vi "FrontPanelToIni.vi"(8 "ErrorArray In":errorcluster[](array[cluster])) -> (0 "ErrorArray Out":errorcluster[](array[cluster]))   [LabVIEW 2014, in "Framework.lvlib"]
uses:
  Framework.lvlib
  <vilib>/Utility/config.llb/Config Data RefNum.ctl
  Config_class/Config.lvclass/Config.ctl
  TypeDefs/clInitParams.ctl
  Config_class/Typedefs/eLogLvl.ctl
  Config_class/Accessors/Read ConfigFilePath.vi
  Config_class/Read Logging.vi
  Config_class/Accessors/Read PARTF Root Directory.vi
  <vilib>/Utility/error.llb/Error Cluster From Error Code.vi
  <vilib>/ErrorRing/Error Ring.xnode
  <userlib>/NIST/NISTErrorLib/NISTErrorLib.lvlib
  <vilib>/Utility/config.llb/NI_LVConfig.lvlib
  Config_class/Config.lvclass
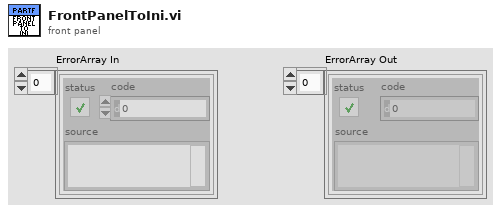
[diagram p1: front panel]
types:
  T1 = typedef "NI_LVConfig.lvlib/Config Data RefNum.ctl" = refnum<k1>
  T2 = typedef "Framework.lvlib/clInitParams.ctl" = cluster{"RowHdrs":string[], "ColHdrs":string[], "DefaultParams":string[][]}
  T3 = typedef "Framework.lvlib/clFrontPanelControlRefs.ctl" = cluster{"TestFilePathRef":refnum<vi>, "BusNumberRef":refnum<vi>, "NumberOfBusesRef":refnum<vi>, "EvtTypeRef":refnum<vi>, "EvtParamsRef":refnum<vi>, "EvtConfigRef":refnum<vi>, "StartTimeRef":refnum<vi>, "EndTimeRef":refnum<vi>, "PmuImpairTypeRef":refnum<vi>, "PmuImpairParamsRef":refnum<vi>, "NetImpairParamsRef":refnum<vi>, "FlagImpairTypeRef":refnum<vi>, "FlagImpairParamsRef":refnum<vi>, "NetImpairTypeRef":refnum<vi>, "OutputFileType":refnum<vi>, "PmuImpairConfigRef":refnum<vi>, "AppTypeRef":refnum<vi>, "ScriptPathRef":refnum<vi>, "ShowPanels?":refnum<vi>}
  T4 = typedef "Framework.lvlib/clEventConfig.ctl" = cluster{"UTC Time 0":timestamp, "Nominal Frequency":u16, "Reporting Rate":u16, "Fsamp":u32, "PosSeq":bool}
  T5 = typedef "PmuImpairPlugins.lvlib/PmuImpairPluginBase.lvclass/clImpairConfig.ctl" = cluster{"FilterType":string, "bPosSeq":bool}
  T6 = typedef "Framework.lvlib/Config.lvclass/eLogLvl.ctl" = enum16{"Normal", "Verbose", "None"}
  T7 = cluster{"pathRootDir":path, "OutDir":string, "ScriptDir":string, "TestDir":string}
  T8 = typedef "Framework.lvlib/Config.lvclass/Logging.ctl" = cluster{"eLogLvl":T6, "Log File Path":path, "btnLogFile":bool}
  T9 = typedef "Framework.lvlib/Config.lvclass/RootDir.ctl" = cluster{"pathRootDir":path, "btnOutPath":bool, "OutDir":string, "btnOpenOutputDir":bool, "ScriptDir":string, "btnOpenScriptDir":bool, "TestDir":string, "btnOpenTestDir":bool}
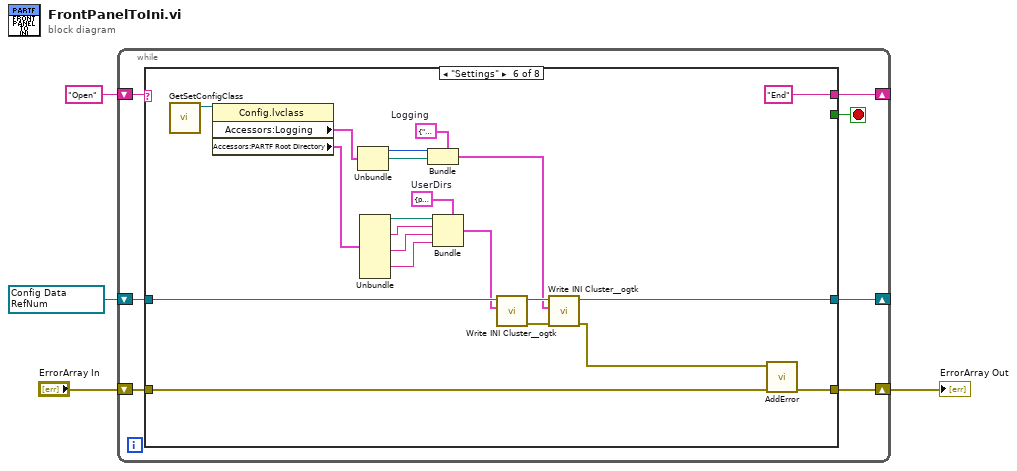
[diagram p0: block diagram]
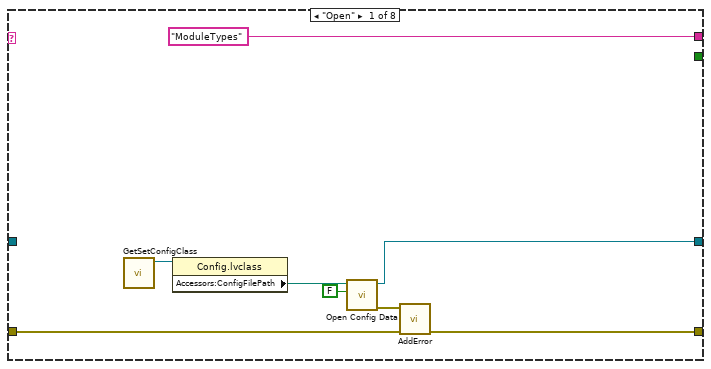
[diagram p2: hidden frame]
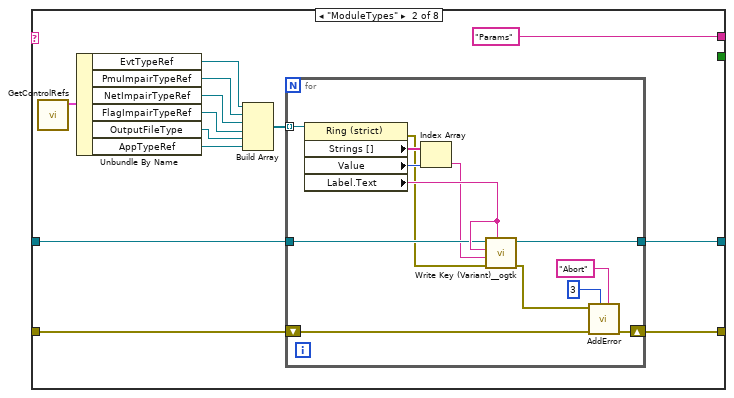
[diagram p3: hidden frame]
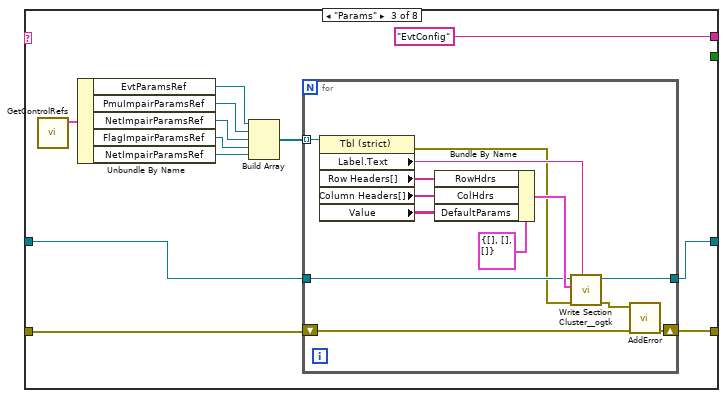
[diagram p4: hidden frame]
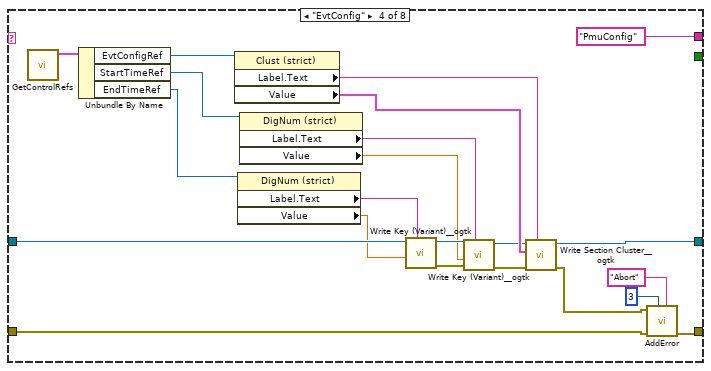
[diagram p5: hidden frame]
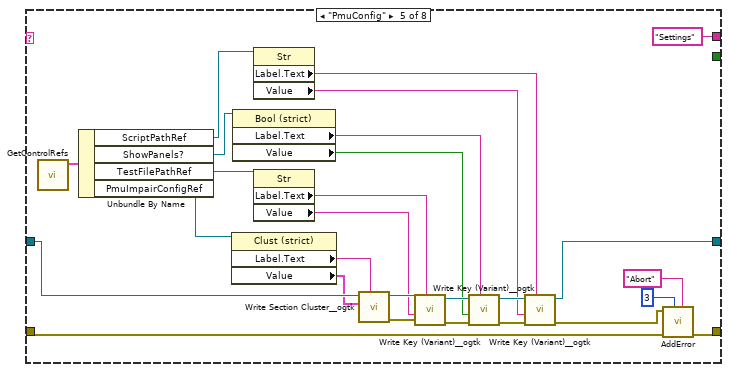
[diagram p6: hidden frame]
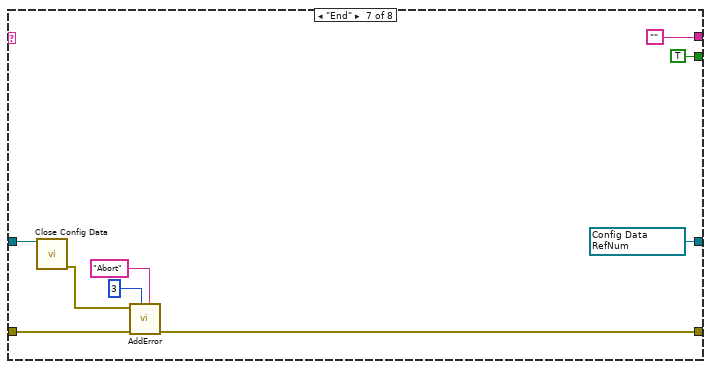
[diagram p7: hidden frame]
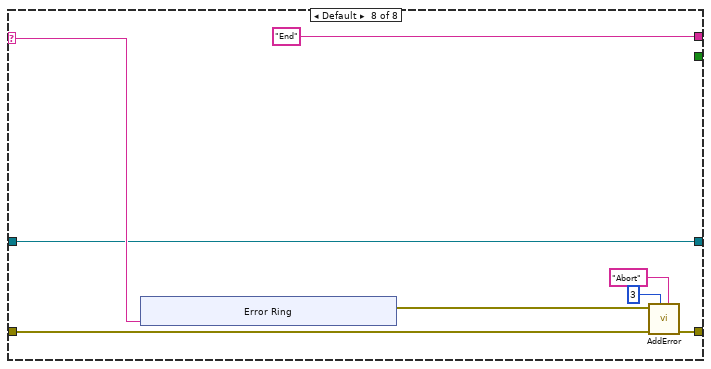
[diagram p8: hidden frame]
diagram:
  w1 = T1 refnum items=["config data"] ("refnum")
  n1 = while {
    shift-right: [w9] -> w2
    shift-left: "ErrorArray In" -> [w10]
    shift-right: [w8] -> _
    shift-left: w1 -> [w6]
    shift-right: [w7] -> _
    shift-left: "Open" -> [w11]
    stop <- w5 stop-if-true
    n2 = case shown="\"Settings\"" w11 {
      selector: w11 -> [_ _ _ _ _ _ _ w157]
      tunnel: w10 -> [w14 w23 w47 w71 w96 w122 w145 w153]
      tunnel: [w13 w22 w48 w75 w98 w123 w144 w152] -> w9
      tunnel: [w16 w21 w49 w76 w93 w124 w141 w150] -> w8
      tunnel: ["ModuleTypes" "Params" "EvtConfig" "PmuConfig" "Settings" "End" "" "End"] -> w7
      tunnel: w6 -> [_ w24 w50 w84 w116 w129 w147 w150]
      tunnel: [_ _ _ _ _ _ TRUE _] -> w5
      frame "Open" {
        n3 = call "GetSetConfigClass.vi"() -> ("Ref out"=w19:refnum<class "Config.lvclass">)  [unwired: 11 in]
        n4 = property class="Config.lvclass"(reference=w19) -> ("Accessors:ConfigFilePath"=w18:path)  [unwired: 1 in, 2 out]
        n5 = call <vilib>:"Open Config Data.vi"("create file if necessary (T)"=FALSE, "configuration file path"=w18) -> ("error out"=w15:errorcluster, "refnum"=w16:T1)  [unwired: 7 in, 1 out]
        n6 = call <userlib>:"AddError.vi"("ErrorArray"=w14, "error in (no error)"=w15) -> ("ErrorArray"=w13:errorcluster[])  [unwired: 8 in, 1 out]
      }
      frame "ModuleTypes" {
        n7 = call "GetControlRefs.vi"() -> ("clControlRefs Out"=w32:T3)  [unwired: 11 in]
        n8 = Unbundle By Name(w32) -> ("EvtTypeRef"=w26:refnum<vi>, "PmuImpairTypeRef"=w27:refnum<vi>, "NetImpairTypeRef"=w28:refnum<vi>, "FlagImpairTypeRef"=w29:refnum<vi>, "OutputFileType"=w30:refnum<vi>, "AppTypeRef"=w31:refnum<vi>)
        n9 = Build Array(w26, w27, w28, w29, w30, w31) -> (w25:refnum<vi>[])
        n10 = for {
          tunnel: w25 -> [w45] mode=indexing
          tunnel: w24 -> [w43]
          shift-right: [w36] -> w22
          shift-left: w23 -> [w37]
          tunnel: [w35] -> w21
          n11 = property class="Ring (strict)"(reference=w45) -> (error out=w33:errorcluster, "Strings []"=w42:string[], "Value"=w41:u16, "Label.Text"=w44:string)  [unwired: 1 in, 1 out]
          n12 = Index Array(array=w42, index=w41) -> (element=w40:string)
          n13 = call <userlib>:"Write Key (Variant)__ogtk.vi"("section"=w44, "error in (no error)"=w33, "key-value"=w40, "key (optional)"=w44, "refnum"=w43) -> ("error out"=w34:errorcluster, "refnum out"=w35:T1)  [unwired: 5 in]
          n14 = call <userlib>:"AddError.vi"("Severity"="Abort", "Priority"=u8 3, "ErrorArray"=w37, "error in (no error)"=w34) -> ("ErrorArray"=w36:errorcluster[])  [unwired: 6 in, 1 out]
        }
      }
      frame "Params" {
        n15 = call "GetControlRefs.vi"() -> ("clControlRefs Out"=w52:T3)  [unwired: 11 in]
        n16 = Unbundle By Name(w52) -> ("EvtParamsRef"=w57:refnum<vi>, "PmuImpairParamsRef"=w56:refnum<vi>, "NetImpairParamsRef"=w55:refnum<vi>, "FlagImpairParamsRef"=w54:refnum<vi>, "NetImpairParamsRef"=w53:refnum<vi>)
        n17 = Build Array(w57, w56, w55, w54, w53) -> (w51:refnum<vi>[])
        n18 = for {
          tunnel: w51 -> [w70] mode=indexing
          tunnel: w50 -> [w63]
          tunnel: [w62] -> w49
          shift-right: [w61] -> w48
          shift-left: w47 -> [w60]
          n19 = property class="Tbl (strict)"(reference=w70) -> (error out=w58:errorcluster, "Label.Text"=w65:string, "Row Headers[]"=w68:string[], "Column Headers[]"=w67:string[], "Value"=w66:string[][])  [unwired: 1 in, 1 out]
          n20 = Bundle By Name(cluster=T2 {"RowHdrs"=[], "ColHdrs"=[], "DefaultParams"=[]} ("ParamsHdrs"), "RowHdrs"=w68, "ColHdrs"=w67, "DefaultParams"=w66) -> (w64:T2)
          n21 = call <userlib>:"Write Section Cluster__ogtk.vi"("section (optional)"=w65, "error in (no error)"=w58, "Section Formatted Cluster"=w64, "refnum"=w63) -> ("error out"=w59:errorcluster, "dup refnum"=w62:T1)  [unwired: 6 in]
          n22 = call <userlib>:"AddError.vi"("ErrorArray"=w60, "error in (no error)"=w59) -> ("ErrorArray"=w61:errorcluster[])  [unwired: 8 in, 1 out]
        }
      }
      frame "EvtConfig" {
        n23 = call "GetControlRefs.vi"() -> ("clControlRefs Out"=w91:T3)  [unwired: 11 in]
        n24 = Unbundle By Name(w91) -> ("EvtConfigRef"=w90:refnum<vi>, "StartTimeRef"=w89:refnum<vi>, "EndTimeRef"=w88:refnum<vi>)
        n25 = property class="Clust (strict)"(reference=w90) -> ("Label.Text"=w79:string, "Value"=w78:T4)  [unwired: 1 in, 2 out]
        n26 = property class="DigNum (strict)"(reference=w88) -> ("Label.Text"=w85:string, "Value"=w83:dbl)  [unwired: 1 in, 2 out]
        n27 = property class="DigNum (strict)"(reference=w89) -> ("Label.Text"=w82:string, "Value"=w81:dbl)  [unwired: 1 in, 2 out]
        n28 = call <userlib>:"Write Key (Variant)__ogtk.vi"("section"=w85, "key-value"=w83, "refnum"=w84) -> ("error out"=w87:errorcluster, "refnum out"=w86:T1)  [unwired: 7 in]
        n29 = call <userlib>:"Write Key (Variant)__ogtk.vi"("section"=w82, "error in (no error)"=w87, "key-value"=w81, "refnum"=w86) -> ("error out"=w80:errorcluster, "refnum out"=w77:T1)  [unwired: 6 in]
        n30 = call <userlib>:"Write Section Cluster__ogtk.vi"("section (optional)"=w79, "error in (no error)"=w80, "Section Formatted Cluster"=w78, "refnum"=w77) -> ("error out"=w72:errorcluster, "dup refnum"=w76:T1)  [unwired: 6 in]
        n31 = call <userlib>:"AddError.vi"("Severity"="Abort", "Priority"=u8 3, "ErrorArray"=w71, "error in (no error)"=w72) -> ("ErrorArray"=w75:errorcluster[])  [unwired: 6 in, 1 out]
      }
      frame "PmuConfig" {
        n32 = call "GetControlRefs.vi"() -> ("clControlRefs Out"=w118:T3)  [unwired: 11 in]
        n33 = Unbundle By Name(w118) -> ("ScriptPathRef"=w111:refnum<vi>, "ShowPanels?"=w112:refnum<vi>, "TestFilePathRef"=w113:refnum<vi>, "PmuImpairConfigRef"=w117:refnum<vi>)
        n34 = property class="Clust (strict)"(reference=w117) -> ("Label.Text"=w115:string, "Value"=w114:T5)  [unwired: 1 in, 2 out]
        n35 = property class="Bool (strict)"(reference=w112) -> ("Label.Text"=w102:string, "Value"=w101:bool)  [unwired: 1 in, 2 out]
        n36 = property class="Str"(reference=w111) -> ("Label.Text"=w100:string, "Value"=w99:string)  [unwired: 1 in, 2 out]
        n37 = property class="Str"(reference=w113) -> ("Label.Text"=w104:string, "Value"=w103:string)  [unwired: 1 in, 2 out]
        n38 = call <userlib>:"Write Section Cluster__ogtk.vi"("section (optional)"=w115, "Section Formatted Cluster"=w114, "refnum"=w116) -> ("error out"=w110:errorcluster, "dup refnum"=w109:T1)  [unwired: 7 in]
        n39 = call <userlib>:"Write Key (Variant)__ogtk.vi"("section"=w104, "error in (no error)"=w110, "key-value"=w103, "refnum"=w109) -> ("error out"=w105:errorcluster, "refnum out"=w106:T1)  [unwired: 6 in]
        n40 = call <userlib>:"Write Key (Variant)__ogtk.vi"("section"=w102, "error in (no error)"=w105, "key-value"=w101, "refnum"=w106) -> ("error out"=w108:errorcluster, "refnum out"=w107:T1)  [unwired: 6 in]
        n41 = call <userlib>:"Write Key (Variant)__ogtk.vi"("section"=w100, "error in (no error)"=w108, "key-value"=w99, "refnum"=w107) -> ("error out"=w97:errorcluster, "refnum out"=w93:T1)  [unwired: 6 in]
        n42 = call <userlib>:"AddError.vi"("Severity"="Abort", "Priority"=u8 3, "ErrorArray"=w96, "error in (no error)"=w97) -> ("ErrorArray"=w98:errorcluster[])  [unwired: 6 in, 1 out]
      }
      frame "Settings" {
        w120 = cluster{"eLogLvl":T6, "Log File Path":path} {"eLogLvl"=enum."Normal", "Log File Path"=path ""}  # Logging
        w138 = T7 {"pathRootDir"=path "", "OutDir"="", "ScriptDir"="", "TestDir"=""}  # UserDirs
        n43 = call "GetSetConfigClass.vi"() -> ("Ref out"=w139:refnum<class "Config.lvclass">)  [unwired: 11 in]
        n44 = property class="Config.lvclass"(reference=w139) -> ("Accessors:Logging"=w130:T8, "Accessors:PARTF Root Directory"=w133:T9)  [unwired: 1 in, 2 out]
        n45 = Unbundle(w130) -> ("eLogLvl"=w131:T6, "Log File Path"=w132:path)  [unwired: 1 out]
        n46 = Unbundle(w133) -> ("pathRootDir"=w134:path, "OutDir"=w135:string, "ScriptDir"=w136:string, "TestDir"=w137:string)  [unwired: 4 out]
        n47 = Bundle(cluster=w120, "eLogLvl"=w131, "Log File Path"=w132) -> (w125:cluster{"eLogLvl":T6, "Log File Path":path})
        n48 = Bundle(cluster=w138, "pathRootDir"=w134, "OutDir"=w135, "ScriptDir"=w136, "TestDir"=w137) -> (w128:T7)
        n49 = call <userlib>:"Write INI Cluster__ogtk.vi"("INI Fomatted Cluster"=w128, "refnum"=w129) -> ("error out"=w127:errorcluster, "dup refnum"=w126:T1)  [unwired: 8 in]
        n50 = call <userlib>:"Write INI Cluster__ogtk.vi"("error in (no error)"=w127, "INI Fomatted Cluster"=w125, "refnum"=w126) -> ("error out"=w121:errorcluster, "dup refnum"=w124:T1)  [unwired: 7 in]
        n51 = call <userlib>:"AddError.vi"("ErrorArray"=w122, "error in (no error)"=w121) -> ("ErrorArray"=w123:errorcluster[])  [unwired: 8 in, 1 out]
      }
      frame "End" {
        w141 = T1 refnum items=["config data"] ("dup refnum")
        n52 = call <vilib>:"Close Config Data.vi"("refnum"=w147) -> ("error out"=w146:errorcluster)  [unwired: 9 in, 1 out]
        n53 = call <userlib>:"AddError.vi"("Severity"="Abort", "Priority"=u8 3, "ErrorArray"=w145, "error in (no error)"=w146) -> ("ErrorArray"=w144:errorcluster[])  [unwired: 6 in, 1 out]
      }
      frame Default {
        n54 = xnode "Error Ring"("parameter 0"=w157) -> ("error out"=w156:errorcluster)
        n55 = call <userlib>:"AddError.vi"("Severity"="Abort", "Priority"=u8 3, "ErrorArray"=w153, "error in (no error)"=w156) -> ("ErrorArray"=w152:errorcluster[])  [unwired: 6 in, 1 out]
      }
    }
  }
  "ErrorArray Out" <- w2
